vi "ParseArray.vi"(8 "error in (no error)":errorcluster, 10 "Index In":i32, 11 "JSON String":string) -> (0 "error out":errorcluster, 2 "Index Out":i32, 3 "JSON Tree":variant)   [LabVIEW 2013, in "i3-json.lvlib"]
doc: "Use this template to build a VI to use as a subVI."
uses:
  i3-json.lvlib
  JSON Types/JSON Type.ctl
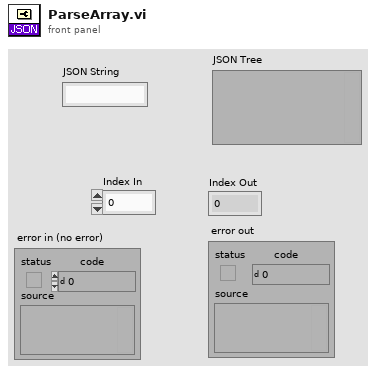
[diagram p1: front panel]
types:
  T1 = typedef "i3-json.lvlib/JSON Type.ctl" = enum8{"JSON Compatible", "JSON Array", "JSON Object", "JSON Null", "Double", "String", "Boolean", "Unknown", "Data JSON string"}
  T2 = typedef "i3-json.lvlib/Token.ctl" = enum16{"NONE", "CURLY_OPEN", "CURLY_CLOSE", "SQUARED_OPEN", "SQUARED_CLOSE", "COLON", "COMMA", "STRING", "NUMBER", "TRUE", "FALSE", "NULL"}
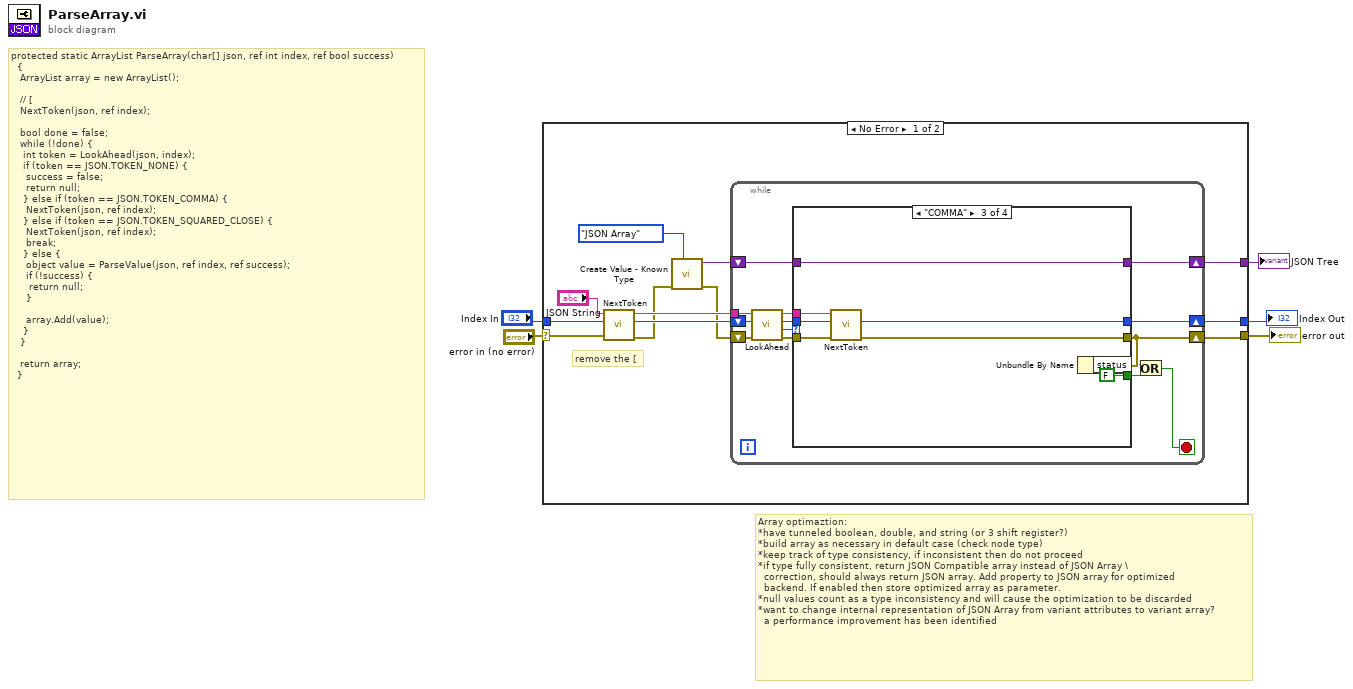
[diagram p0: block diagram]
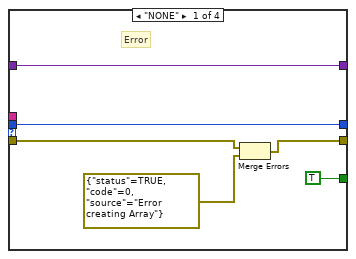
[diagram p2: hidden frame]
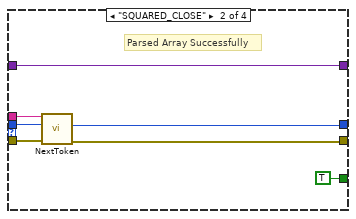
[diagram p3: hidden frame]
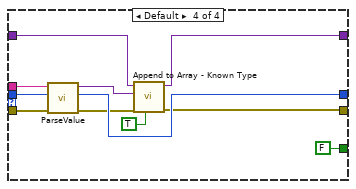
[diagram p4: hidden frame]
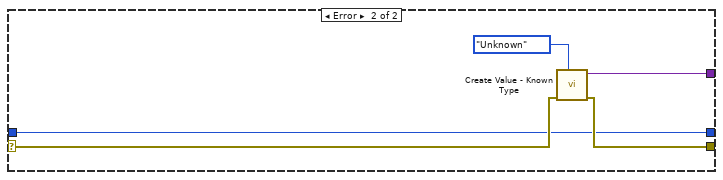
[diagram p5: hidden frame]
diagram:
  # "Array optimaztion:\n*have tunneled boolean, double, and string (or 3 shift register?)\n*build array as necessary in default case (check node type)\n*keep track of type consistency, if inconsistent then do not proceed\n*if type fully consistent, return JSON Compatible array instead of JSON Array \\\n  correction, should always return JSON array. Add property to JSON array for optimized\n  backend. If enabled then store optimized array as parameter.\n*null values count as a type inconsistency and will cause the optimization to be discarded\n*want to change internal representation of JSON Array from variant attributes to variant array?\n  a performance improvement has been identified"
  # "protected static ArrayList ParseArray(char[] json, ref int index, ref bool success)\n\t\t{\n\t\t\tArrayList array = new ArrayList();\n\n\t\t\t// [\n\t\t\tNextToken(json, ref index);\n\n\t\t\tbool done = false;\n\t\t\twhile (!done) {\n\t\t\t\tint token = LookAhead(json, index);\n\t\t\t\tif (token == JSON.TOKEN_NONE) {\n\t\t\t\t\tsuccess = false;\n\t\t\t\t\treturn null;\n\t\t\t\t} else if (token == JSON.TOKEN_COMMA) {\n\t\t\t\t\tNextToken(json, ref index);\n\t\t\t\t} else if (token == JSON.TOKEN_SQUARED_CLOSE) {\n\t\t\t\t\tNextToken(json, ref index);\n\t\t\t\t\tbreak;\n\t\t\t\t} else {\n\t\t\t\t\tobject value = ParseValue(json, ref index, ref success);\n\t\t\t\t\tif (!success) {\n\t\t\t\t\t\treturn null;\n\t\t\t\t\t}\n\n\t\t\t\t\tarray.Add(value);\n\t\t\t\t}\n\t\t\t}\n\n\t\t\treturn array;\n\t\t}"
  n1 = case shown="No Error" "error in (no error)" {
    selector: "error in (no error)" -> [w17 w67]
    tunnel: [w6 w66] -> w4
    tunnel: "Index In" -> [w16 w65]
    tunnel: [w8 w65] -> w2
    tunnel: [w7 w64] -> w1
    frame No Error {
      # "remove the ["
      n2 = call "NextToken.vi"("error in (no error)"=w17, "Index In"=w16, "JSON String"="JSON String") -> ("error out"=w12:errorcluster, "Index Out"=w14:i32, "JSON String Passthrough"=w13:string)  [unwired: 4 in, 1 out]
      n3 = call "Create Value - Known Type.vi"("JSON Type"=JSON_Type."JSON Array", "error in (no error)"=w12) -> ("error out"=w11:errorcluster, "JSON Tree"=w10:variant)  [unwired: 8 in]
      n4 = while {
        shift-right: [w24] -> w8
        shift-left: w14 -> [w30]
        tunnel: w13 -> [w29]
        shift-right: [w23] -> w7
        shift-left: w10 -> [w22]
        shift-right: [w19] -> w6
        shift-left: w11 -> [w31]
        stop <- w20 stop-if-true
        n5 = call "LookAhead.vi"("error in (no error)"=w31, "Index"=w30, "JSON String"=w29) -> ("error out"=w27:errorcluster, "TOKEN"=w28:T2, "Index Passthrough"=w26:i32, "JSON String Passthrough"=w25:string)  [unwired: 4 in]
        n6 = case shown="\"COMMA\"" w28 {
          tunnel: w27 -> [w33 w44 w49 w62]
          tunnel: [TRUE TRUE FALSE FALSE] -> w21
          tunnel: w26 -> [w36 w43 w50 w61]
          tunnel: w25 -> [_ w42 w51 w60]
          tunnel: [w36 w40 w47 w59] -> w24
          tunnel: [w35 w39 w46 w53] -> w23
          tunnel: w22 -> [w35 w39 w46 w54]
          tunnel: [w34 w41 w48 w52] -> w19
          frame "NONE" {
            # "Error"
            n7 = Merge Errors(w33, errorcluster {"status"=TRUE, "code"=0, "source"="Error creating Array"} ("error out")) -> (w34:errorcluster)
          }
          frame "SQUARED_CLOSE" {
            # "Parsed Array Successfully"
            n8 = call "NextToken.vi"("error in (no error)"=w44, "Index In"=w43, "JSON String"=w42) -> ("error out"=w41:errorcluster, "Index Out"=w40:i32)  [unwired: 4 in, 2 out]
          }
          frame "COMMA" {
            n9 = call "NextToken.vi"("error in (no error)"=w49, "Index In"=w50, "JSON String"=w51) -> ("error out"=w48:errorcluster, "Index Out"=w47:i32)  [unwired: 4 in, 2 out]
          }
          frame Default {
            n10 = call "ParseValue.vi"("error in (no error)"=w62, "Index In"=w61, "JSON String"=w60) -> ("error out"=w57:errorcluster, "Index Out"=w59:i32, "JSON Tree"=w56:variant)  [unwired: 6 in]
            n11 = call "Append to Array - Known Type.vi"("Add Parameter as JSON Tree?"=TRUE, "error in (no error)"=w57, "Value"=w56, "JSON Tree in (JSON Array)"=w54) -> ("error out"=w52:errorcluster, "JSON Tree out (JSON Array)"=w53:variant)  [unwired: 6 in]
          }
        }
        n12 = Unbundle By Name(w19) -> ("status"=w18:bool)
        n13 = Or(x=w18, y=w21) -> (x .or. y?=w20:bool)
      }
    }
    frame Error {
      n14 = call "Create Value - Known Type.vi"("JSON Type"=JSON_Type."Unknown", "error in (no error)"=w67) -> ("error out"=w66:errorcluster, "JSON Tree"=w64:variant)  [unwired: 8 in]
    }
  }
  "error out" <- w4
  "Index Out" <- w2
  "JSON Tree" <- w1
